vi "LogEvent.vi"(8 "error in (no error)":errorcluster, 10 "Text Message to Log":string, 11 "object in":refnum<class "EventLogger_Actor.lvclass">) -> (0 "error out":errorcluster, 3 "object out":refnum<class "EventLogger_Actor.lvclass">)   [LabVIEW 2014, in "EventLogger_Actor.lvlib" / "EventLogger_Actor.lvclass"]
uses:
  EventLogger_Actor.lvclass
  EventLogger_Actor.lvclass/EventLogger_Actor.ctl
  <userlib>/_OpenG.lib/string/string.llb/Trim Whitespace (String)__ogtk.vi
panel:
  # "BSD 2-Clause License\n\nCopyright (c) 2018, Ajay www.digiajay.com\nAll rights reserved.\n\nRedistribution and use in source and binary forms, with or without\nmodification, are permitted provided that the following conditions are met:\n\n* Redistributions of source code must retain the above copyright notice, this\n  list of conditions and the following disclaimer.\n\n* Redistributions in binary form must reproduce the above copyright notice,\n  this list of conditions and the following disclaimer in the documentation\n  and/or other materials provided with the distribution.\n\nTHIS SOFTWARE IS PROVIDED BY THE COPYRIGHT HOLDERS AND CONTRIBUTORS \"AS IS\"\nAND ANY EXPRESS OR IMPLIED WARRANTIES, INCLUDING, BUT NOT LIMITED TO, THE\nIMPLIED WARRANTIES OF MERCHANTABILITY AND FITNESS FOR A PARTICULAR PURPOSE ARE\nDISCLAIMED. IN NO EVENT SHALL THE COPYRIGHT HOLDER OR CONTRIBUTORS BE LIABLE\nFOR ANY DIRECT, INDIRECT, INCIDENTAL, SPECIAL, EXEMPLARY, OR CONSEQUENTIAL\nDAMAGES (INCLUDING, BUT NOT LIMITED TO, PROCUREMENT OF SUBSTITUTE GOODS OR\nSERVICES; LOSS OF USE, DATA, OR PROFITS; OR BUSINESS INTERRUPTION) HOWEVER\nCAUSED AND ON ANY THEORY OF LIABILITY, WHETHER IN CONTRACT, STRICT LIABILITY,\nOR TORT (INCLUDING NEGLIGENCE OR OTHERWISE) ARISING IN ANY WAY OUT OF THE USE\nOF THIS SOFTWARE, EVEN IF ADVISED OF THE POSSIBILITY OF SUCH DAMAGE."
  # "Connector Pane"
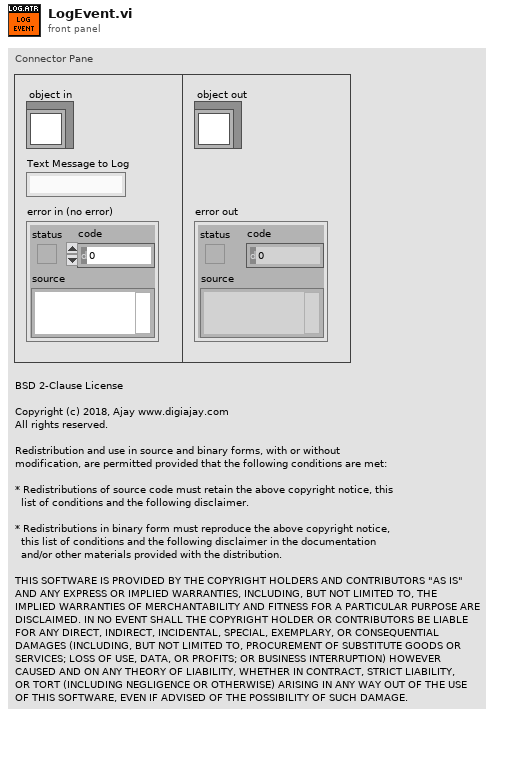
[diagram p1: front panel]
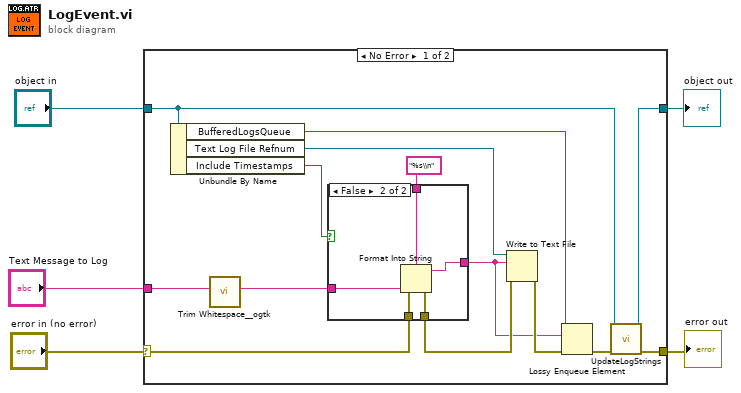
[diagram p0: block diagram]
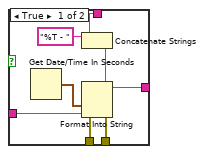
[diagram p2: hidden frame]
diagram:
  n1 = case shown="No Error" "error in (no error)" {
    selector: "error in (no error)" -> [w17 w34]
    tunnel: [w8 w34] -> w4
    tunnel: [w7 w33] -> w2
    tunnel: "object in" -> [w6 w33]
    tunnel: "Text Message to Log" -> [w15 _]
    frame No Error {
      n2 = Unbundle By Name(w6) -> ("BufferedLogsQueue"=w9:refnum<queue>, "Text Log File Refnum"=w12:refnum<file>, "Include Timestamps"=w13:bool)
      n3 = call-poly <userlib>:"Trim Whitespace__ogtk.vi"("String in"=w15) -> ("String out"=w14:string)  [unwired: 6 in]
      n4 = case shown="False" w13 {
        tunnel: "%s\\n" ("format string") -> [w27 w28]
        tunnel: w17 -> [w25 w32]
        tunnel: [w24 w31] -> w16
        tunnel: [w23 w30] -> w10
        tunnel: w14 -> [w22 w29]
        frame True {
          n5 = Get Date/Time In Seconds() -> (seconds since 1Jan1904=w26:timestamp)
          n6 = Concatenate Strings("%T - " ("string"), w27) -> (w21:string)
          n7 = Format Into String(format string=w21, error in=w25, w26, w22) -> (resulting string=w23:string, error out=w24:errorcluster)  [unwired: 1 in]
        }
        frame False {
          n8 = Format Into String(format string=w28, error in=w32, w29) -> (resulting string=w30:string, error out=w31:errorcluster)  [unwired: 1 in]
        }
      }
      n9 = Write to Text File(file (use dialog)=w12, text=w10, error in=w16) -> (error out=w19:errorcluster)  [unwired: 1 in, 2 out]
      n10 = Lossy Enqueue Element(queue=w9, element=w10, error in (no error)=w19) -> (error out=w11:errorcluster)  [unwired: 3 out]
      n11 = call "UpdateLogStrings.vi"("error in (no error)"=w11, "object in"=w6) -> ("error out"=w8:errorcluster, "object out"=w7:refnum<class "EventLogger_Actor.lvclass">)  [unwired: 8 in]
    }
    frame Error {
    }
  }
  "error out" <- w4
  "object out" <- w2
